vi "AB_Engine_InteropAssembly_ProtoDefined.vi"(0 "Parser":refnum<k24>, 1 "2011CompatibilityMode":bool, 5 "Build Interop Assembly for .NET 2.0":bool, 7 "ClassInfo":T3[](array[typedef]), 9 "ExportAssemblyVIinfo":T5[](array[typedef]), 11 "error in":errorcluster) -> (4 "Parser Out":refnum<k24>, 6 "ContainLVClass":bool, 8 "SetVIInformationArray":T2[](array[typedef]), 10 "SetLVCLassInformationArray":T1[](array[typedef]), 15 "error out":errorcluster)   [LabVIEW 2020]
uses:
  e:/builds/penguin/labview/branches/2020/dev/dist/resource/NationalInstruments.LabVIEW.Generator.dll
  resource/NationalInstruments.LabVIEW.Generator.dll
  <vilib>/AppBuilder/AB_InteropAssembly_DistVI_Proto_Info.ctl
  <vilib>/AppBuilder/IOStatus.ctl
  <vilib>/AppBuilder/AB_InteropAssembly_DistVI_Class_Info.ctl
  <vilib>/AppBuilder/AB_InteropAssembly_SetVIInformation.ctl
  <vilib>/AppBuilder/AB_InteropAssembly_SetLVClassInformation.ctl
panel:
  in  "SetLVCLassInformation":T1
  in  "SetVIInformation":T2
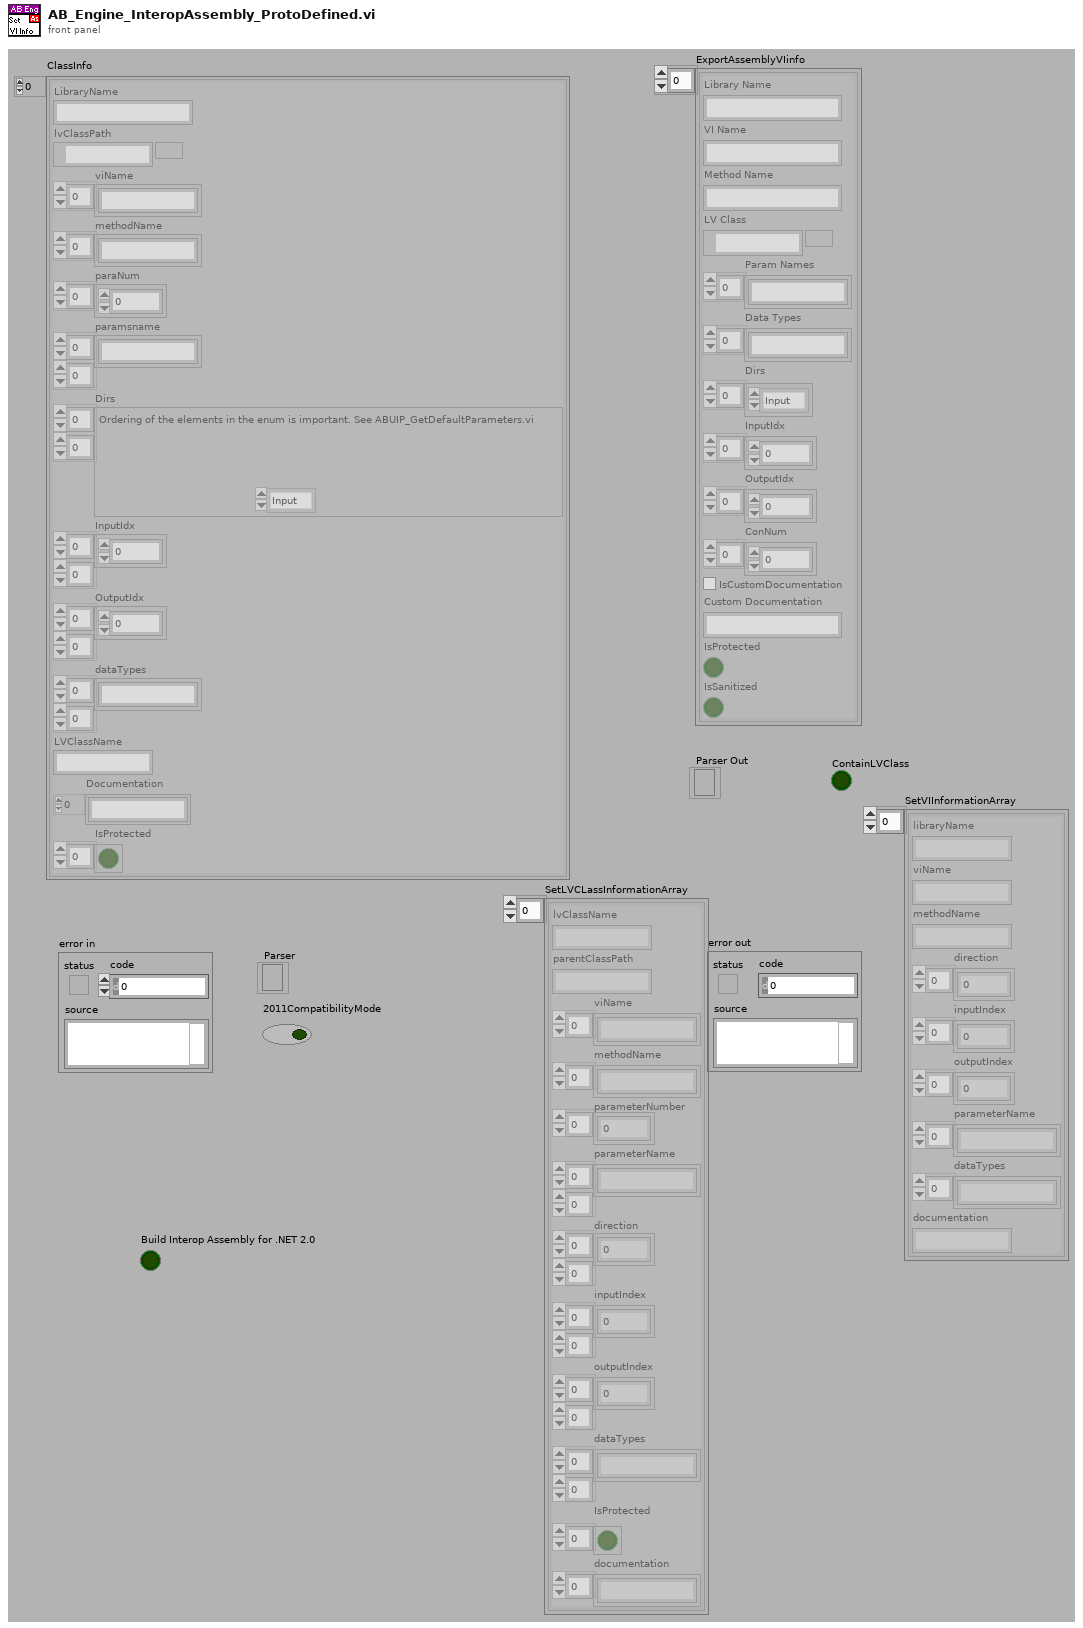
[diagram p1: front panel]
types:
  T1 = typedef "AB_InteropAssembly_SetLVClassInformation.ctl" = cluster{"lvClassName":string, "parentClassPath":string, "viName":string[], "methodName":string[], "parameterNumber":i32[], "parameterName":string[][], "direction":i32[][], "inputIndex":i32[][], "outputIndex":i32[][], "dataTypes":string[][], "IsProtected":bool[], "documentation":string[]}
  T2 = typedef "AB_InteropAssembly_SetVIInformation.ctl" = cluster{"libraryName":string, "viName":string, "methodName":string, "direction":i32[], "inputIndex":i32[], "outputIndex":i32[], "parameterName":string[], "dataTypes":string[], "documentation":string}
  T3 = typedef "AB_InteropAssembly_DistVI_Class_Info.ctl" = cluster{"LibraryName":string, "lvClassPath":path, "viName":string[], "methodName":string[], "paraNum":i32[], "paramsname":string[][], "Dirs":T4[][], "InputIdx":i32[][], "OutputIdx":i32[][], "dataTypes":string[][], "LVClassName":string, "Documentation":string[], "IsProtected":bool[]}
  T4 = typedef "IOStatus.ctl" = enum16{"Input", "Output", "Input/Output", "InputDeleted", "OutputDeleted", "IODeleted", "ErrorClusterIn", "ErrorClusterOut"}
  T5 = typedef "AB_InteropAssembly_DistVI_Proto_Info.ctl" = cluster{"Library Name":string, "VI Name":string, "Method Name":string, "LV Class":path, "Param Names":string[], "Data Types":string[], "Dirs":T4[], "InputIdx":i32[], "OutputIdx":i32[], "ConNum":i8[], "IsCustomDocumentation":bool, "Custom Documentation":string, "IsProtected":bool, "IsSanitized":bool}
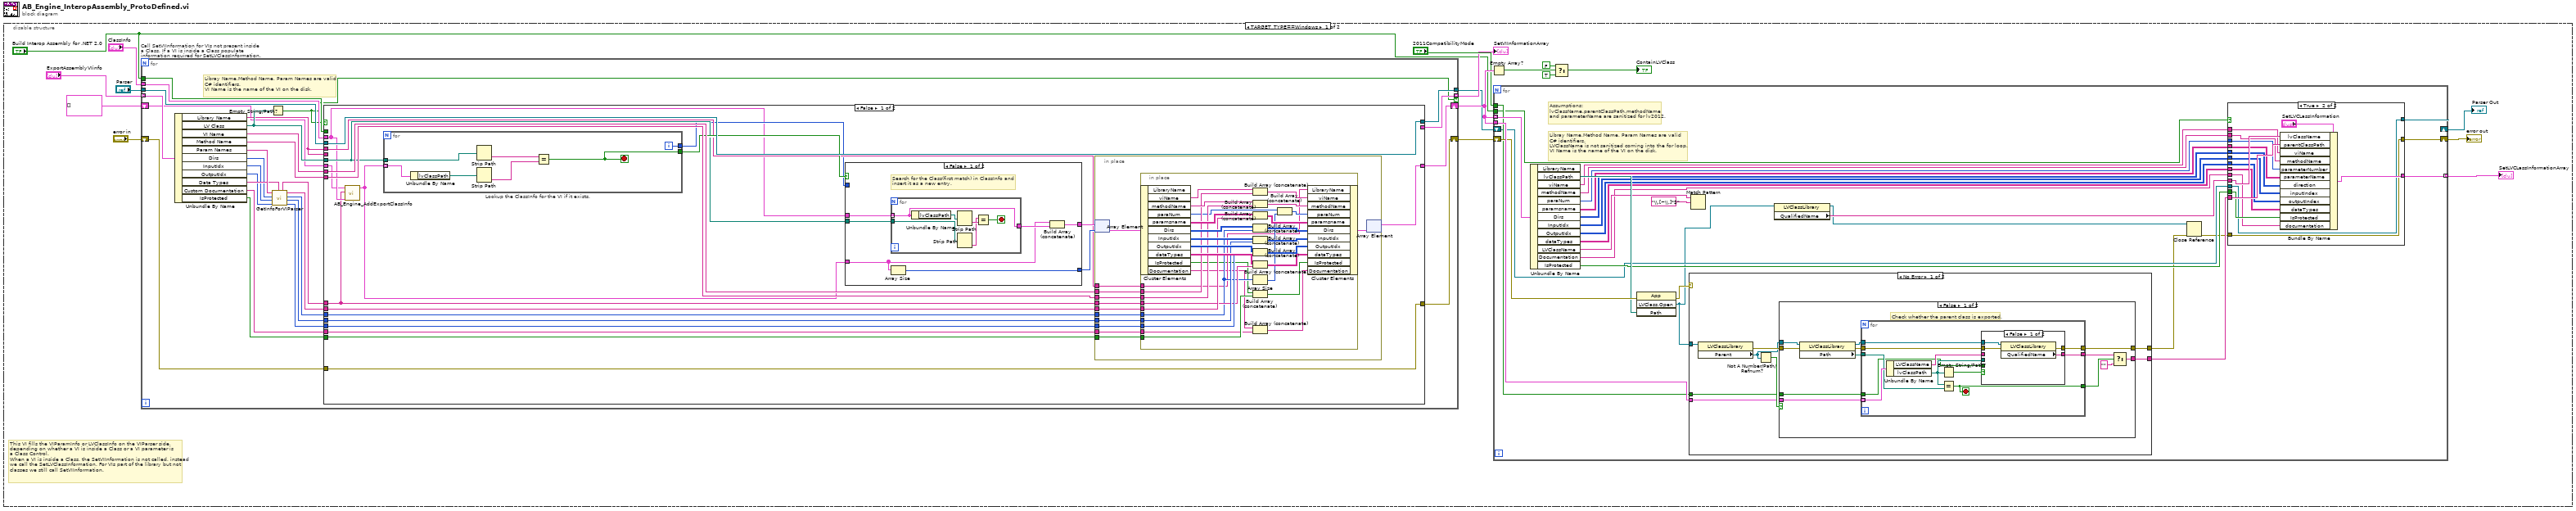
[diagram p0: block diagram]
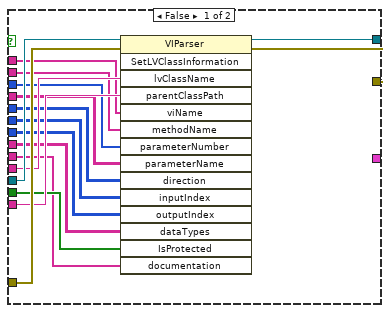
[diagram p2: hidden frame]
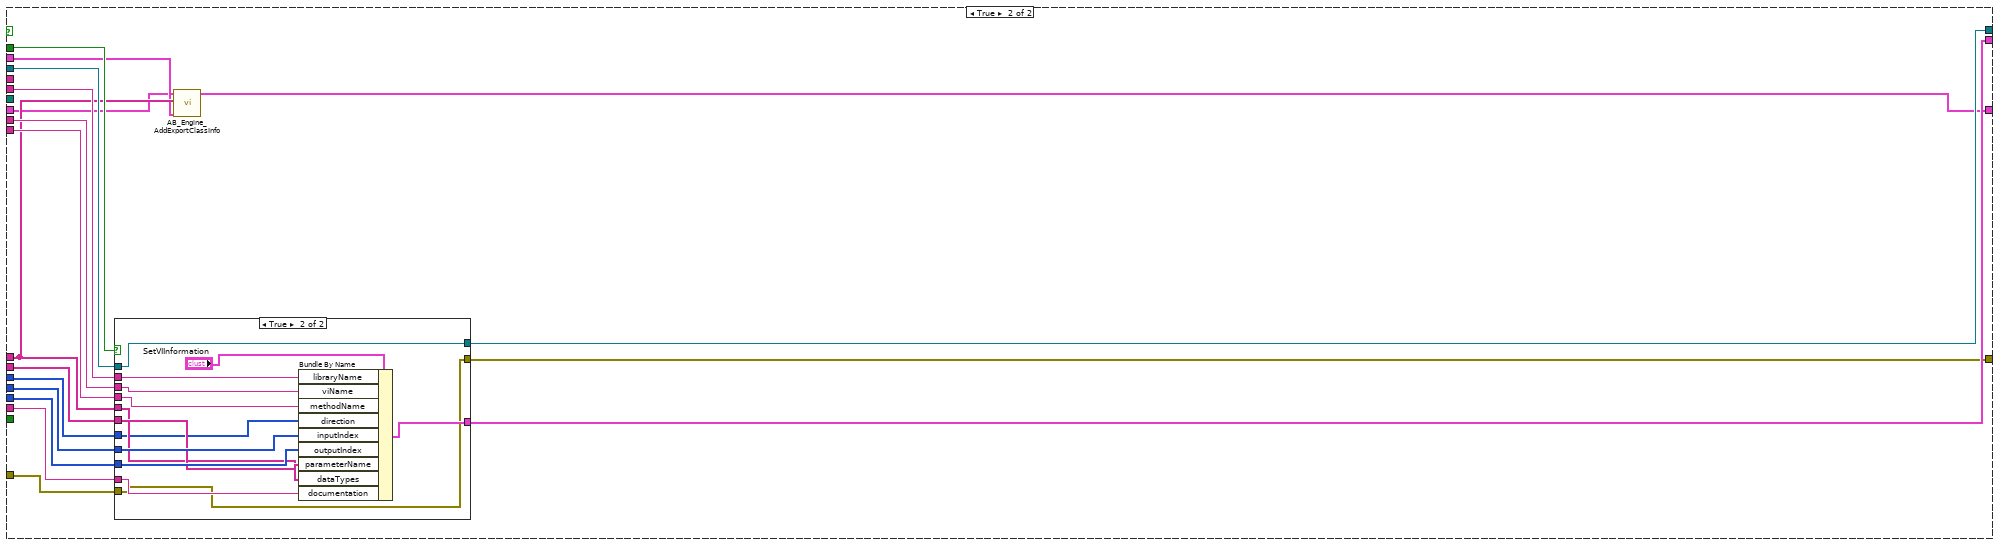
[diagram p7: hidden frame]
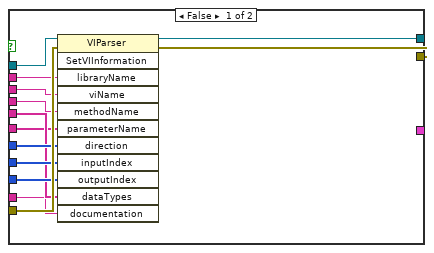
[diagram p8: hidden frame]
diagram:
  n1 = disable-structure shown="TARGET_TYPE==Windows" {
    frame condition #0 (active) {
      # "This VI fills the VIParamInfo or LVClassInfo on the VIParser side,\ndepending on whether a VI is inside a Class or a VI parameter is \na Class Control.\nWhen a VI is inside a Class, the SetVIInformation is not called, instead\nwe call the SetLVClassInformation. For VIs part of the library but not \nclasses we still call SetVIInformation."
      n2 = for "Call SetVIInformation for VIs not present inside a Class. If a VI is inside a Class populate information required for SetLVClassInformation." {
        tunnel: "ExportAssemblyVIinfo" -> [w144] mode=indexing
        tunnel: "Parser" -> [w143]
        shift-right: [w139] -> w15
        shift-left: "error in" -> [w140]
        shift-right: [w141] -> w9
        shift-left: T3[] [] -> [w118]
        tunnel: [w136] -> w2
        tunnel: "ClassInfo" -> [w135]
        tunnel: [w121] -> w4 mode=indexing if=w119
        tunnel: "Build Interop Assembly for .NET 2.0" -> [w120]
        # "Libray Name,Method Name, Param Names are valid\nC# identifiers.\nVI Name is the name of the VI on the disk."
        n3 = Unbundle By Name(w144) -> ("Library Name"=w134:string, "LV Class"=w137:path, "VI Name"=w138:string, "Method Name"=w142:string, "Param Names"=w132:string[], "Dirs"=w130:T4[], "InputIdx"=w129:i32[], "OutputIdx"=w128:i32[], "Data Types"=w131:string[], "Custom Documentation"=w133:string, "IsProtected"=w122:bool)
        n4 = Empty String/Path?(string/path=w137) -> (empty?=w119:bool)
        n5 = call <vilib>:"GetInfoForVIParser.vi"("Data Types"=w131, "OutputIdx"=w128, "InputIdx"=w129, "Dirs"=w130, "Param Names"=w132) -> ("OutputIdx Out"=w123:i32[], "InputIdx Out"=w124:i32[], "Dirs Out"=w126:T4[], "ParamNames Out"=w125:string[], "DataTypesOut"=w127:string[])
        n6 = case shown="False" w119 {
          tunnel: w143 -> [w157 w237]
          tunnel: w138 -> [w165 w244]
          tunnel: w142 -> [w164 w243]
          tunnel: w125 -> [w163 w239]
          tunnel: w126 -> [w162 w242]
          tunnel: w124 -> [w161 w241]
          tunnel: w123 -> [w160 w240]
          tunnel: w127 -> [w145 w233]
          tunnel: [w158 w234] -> w139
          tunnel: w118 -> [w146 w230]
          tunnel: w137 -> [w153 _]
          tunnel: [w159 w232] -> w141
          tunnel: w140 -> [w158 w236]
          tunnel: [w157 w235] -> w136
          tunnel: w135 -> [w147 w231]
          tunnel: w134 -> [w152 _]
          tunnel: w134 -> [_ w245]
          tunnel: w133 -> [w150 w238]
          tunnel: w122 -> [w151 _]
          tunnel: [_ w247] -> w121
          tunnel: w120 -> [_ w246]
          frame False {
            n7 = call <vilib>:"AB_Engine_AddExportClassInfo.vi"("ClassInfo"=w147, "DataTypes"=w145, "ExportClassInfo"=w146) -> ("ExportClassInfoOut"=w148:T3[])  [unwired: 8 in]
            n8 = for "Lookup the ClassInfo for the VI if it exists." {
              tunnel: w148 -> [w186] mode=indexing
              tunnel: w153 -> [w183]
              tunnel: [w184] -> w156
              tunnel: [w185] -> w149
              i -> [w185]
              stop <- w184 stop-if-true
              n9 = Unbundle By Name(w186) -> ("lvClassPath"=w181:path)
              n10 = Strip Path(path=w183) -> (name=w182:string)  [unwired: 1 out]
              n11 = Strip Path(path=w181) -> (name=w180:string)  [unwired: 1 out]
              n12 = Equal?(x=w182, y=w180) -> (x = y?=w184:bool)
            }
            n13 = case shown="False" w156 {
              tunnel: w148 -> [w167 w179]
              tunnel: [w171 w179] -> w155
              tunnel: [w166 w178] -> w154
              tunnel: w149 -> [_ w178]
              tunnel: w147 -> [w170 _]
              tunnel: w153 -> [w169 _]
              frame False {
                # "Search for the Class(first match) in ClassInfo and \ninsert it as a new entry."
                n14 = for {
                  tunnel: w170 -> [w172] mode=indexing
                  tunnel: w169 -> [w176]
                  tunnel: [w172] -> w168
                  stop <- w177 stop-if-true
                  n15 = Unbundle By Name(w172) -> ("lvClassPath"=w175:path)
                  n16 = Strip Path(path=w175) -> (name=w174:string)  [unwired: 1 out]
                  n17 = Strip Path(path=w176) -> (name=w173:string)  [unwired: 1 out]
                  n18 = Equal?(x=w173, y=w174) -> (x = y?=w177:bool)
                }
                n19 = Array Size(array=w167) -> (size(s)=w166:i32)
                n20 = Build Array (concatenate)(w167, w168) -> (w171:T3[])
              }
              frame True {
              }
            }
            n21 = in-place {
              in-place-border: w165 -> [w197]
              in-place-border: w164 -> [w196]
              in-place-border: w163 -> [w195]
              in-place-border: w162 -> [w194]
              in-place-border: w161 -> [w193]
              in-place-border: w160 -> [w192]
              in-place-border: w145 -> [w191]
              in-place-border: w152 -> [w189]
              in-place-border: w151 -> [w188]
              in-place-border: w150 -> [w187]
              n22 = in-place-array #1(w155, w154) -> (w198:T3)
              n23 = in-place {
                in-place-border: w197 -> [w211]
                in-place-border: w196 -> [w215]
                in-place-border: w195 -> [w214]
                in-place-border: w194 -> [w209]
                in-place-border: w193 -> [w213]
                in-place-border: w192 -> [w212]
                in-place-border: w191 -> [w210]
                in-place-border: w189 -> [w205]
                in-place-border: w188 -> [w203]
                in-place-border: w187 -> [w201]
                n24 = in-place-cluster #2(w198) -> ("viName"=w229:string[], "methodName"=w227:string[], "paraNum"=w208:i32[], "paramsname"=w225:string[][], "Dirs"=w223:T4[][], "InputIdx"=w221:i32[][], "OutputIdx"=w219:i32[][], "dataTypes"=w217:string[][], "IsProtected"=w204:bool[], "Documentation"=w200:string[])  [unwired: 1 out]
                n25 = Build Array (concatenate)(w229, w211) -> (w228:string[])
                n26 = Build Array (concatenate)(w227, w215) -> (w226:string[])
                n27 = Build Array (concatenate)(w225, w214) -> (w224:string[][])
                n28 = Build Array (concatenate)(w223, w209) -> (w222:T4[][])
                n29 = Build Array (concatenate)(w221, w213) -> (w220:i32[][])
                n30 = Build Array (concatenate)(w219, w212) -> (w218:i32[][])
                n31 = Build Array (concatenate)(w217, w210) -> (w216:string[][])
                n32 = Array Size(array=w209) -> (size(s)=w207:i32)
                n33 = Build Array (concatenate)(w204, w203) -> (w202:bool[])
                n34 = Build Array (concatenate)(w200, w201) -> (w199:string[])
                n35 = Build Array (concatenate)(w208, w207) -> (w206:i32[])
                n36 = in-place-cluster #2("LibraryName"=w205, "viName"=w228, "methodName"=w226, "paraNum"=w206, "paramsname"=w224, "Dirs"=w222, "InputIdx"=w220, "OutputIdx"=w218, "dataTypes"=w216, "IsProtected"=w202, "Documentation"=w199) -> (w190:T3)
              }
              n37 = in-place-array #1(w190) -> (w159:T3[])  [unwired: 1 out]
            }
          }
          frame True {
            n38 = case shown="True" w246 {
              tunnel: [_ w272] -> w247
              tunnel: w245 -> [w258 w271]
              tunnel: w244 -> [w257 w270]
              tunnel: w243 -> [w256 w269]
              tunnel: w242 -> [w255 w261]
              tunnel: w241 -> [w254 w268]
              tunnel: w240 -> [w253 w267]
              tunnel: w239 -> [w251 w266]
              tunnel: w233 -> [w252 w265]
              tunnel: w238 -> [w250 w264]
              tunnel: w237 -> [w260 w263]
              tunnel: w236 -> [w259 w262]
              tunnel: [w249 w263] -> w235
              tunnel: [w248 w262] -> w234
              frame False {
                n39 = invoke class="VIParser" method="SetVIInformation"(reference=w260, error in=w259, "libraryName"=w258, "viName"=w257, "methodName"=w256, "parameterName"=w251, "direction"=w255, "inputIndex"=w254, "outputIndex"=w253, "dataTypes"=w252, "documentation"=w250) -> (reference out=w249:refnum<k24>, error out=w248:errorcluster)  [unwired: 1 in, 10 out]
              }
              frame True {
                n40 = Bundle By Name(cluster="SetVIInformation", "libraryName"=w271, "viName"=w270, "methodName"=w269, "direction"=w261, "inputIndex"=w268, "outputIndex"=w267, "parameterName"=w266, "dataTypes"=w265, "documentation"=w264) -> (w272:T2)
              }
            }
            n41 = call <vilib>:"AB_Engine_AddExportClassInfo.vi"("ClassInfo"=w231, "DataTypes"=w233, "ExportClassInfo"=w230) -> ("ExportClassInfoOut"=w232:T3[])  [unwired: 8 in]
          }
        }
      }
      "SetVIInformationArray" <- w4
      n42 = Empty Array?(array=w9) -> (empty?=w14:bool)
      n43 = for {
        tunnel: w9 -> [w47] mode=indexing
        shift-right: [w25] -> w10
        shift-left: w15 -> [w45]
        tunnel: w9 -> [w46]
        shift-right: [w26] -> w8
        shift-left: w2 -> [w24]
        tunnel: "2011CompatibilityMode" -> [w40]
        tunnel: [w39] -> w3 mode=indexing
        tunnel: "Build Interop Assembly for .NET 2.0" -> [w27]
        # "Assumptions:\nlvClassName,parentClassPath,methodName\nand parameterName are sanitized for lv2012."
        # "Libray Name,Method Name, Param Names are valid\nC# identifiers.\nLVClassName is not sanitized coming into the for loop.\nVI Name is the name of the VI on the disk."
        n44 = Unbundle By Name(w47) -> ("lvClassPath"=w44:path, "viName"=w37:string[], "methodName"=w36:string[], "paraNum"=w35:i32[], "paramsname"=w34:string[][], "Dirs"=w33:T4[][], "InputIdx"=w32:i32[][], "OutputIdx"=w31:i32[][], "dataTypes"=w30:string[][], "LVClassName"=w41:string, "Documentation"=w28:string[], "IsProtected"=w29:bool[])  [unwired: 1 out]
        n45 = invoke class="App" method="LVClass.Open"(error in=w45, "Path"=w44) -> (error out=w43:errorcluster, "LVClass.Open"=w22:refnum<vi>)  [unwired: 2 in, 2 out]
        n46 = case shown="No Error" w43 {
          tunnel: w22 -> [w87 _]
          tunnel: [w86 _] -> w21
          tunnel: w46 -> [w82 _]
          tunnel: [w81 _] -> w38
          tunnel: w40 -> [w80 _]
          frame No Error {
            n47 = property class="LVClassLibrary"(reference=w87) -> (error out=w85:errorcluster, "Parent"=w84:refnum<vi>)  [unwired: 1 in, 1 out]
            n48 = Not A Number/Path/Refnum?(number/path/refnum=w84) -> (NaN/Path/Refnum?=w83:bool)
            n49 = case shown="False" w83 {
              tunnel: w84 -> [w98 _]
              tunnel: [w88 w117] -> w86
              tunnel: [w93 _] -> w81
              tunnel: w85 -> [w99 w117]
              tunnel: w82 -> [w97 _]
              tunnel: w80 -> [w91 _]
              frame False {
                # "Check whether the parent class is exported."
                n50 = property class="LVClassLibrary"(reference=w98, error in=w99) -> (reference out=w90:refnum<vi>, error out=w89:errorcluster, "Path"=w96:path)
                n51 = for {
                  tunnel: w97 -> [w110] mode=indexing
                  tunnel: w96 -> [w109]
                  tunnel: [w106] -> w95
                  tunnel: [w103] -> w94
                  tunnel: w91 -> [w104]
                  tunnel: w90 -> [w102]
                  tunnel: w89 -> [w101]
                  tunnel: [w100] -> w88
                  stop <- w106 stop-if-true
                  n52 = Unbundle By Name(w110) -> ("LVClassName"=w107:string, "lvClassPath"=w108:path)
                  n53 = Empty String/Path?(string/path=w108) -> (empty?=w105:bool)
                  n54 = Equal?(x=w108, y=w109) -> (x = y?=w106:bool)
                  n55 = case shown="False" w105 {
                    tunnel: w108 -> [_ _]
                    tunnel: w107 -> [_ w116]
                    tunnel: [w113 w116] -> w103
                    tunnel: w104 -> [_ _]
                    tunnel: w102 -> [w114 _]
                    tunnel: w101 -> [w112 w115]
                    tunnel: [w111 w115] -> w100
                    frame False {
                      n56 = property class="LVClassLibrary"(reference=w114, error in=w112) -> (error out=w111:errorcluster, "QualifiedName"=w113:string)  [unwired: 1 out]
                    }
                    frame True {
                    }
                  }
                }
                n57 = Select(t=w94, s=w95, f="") -> (s? t:f=w93:string)
              }
              frame True {
                # "LVClass does not have a parent Class."
              }
            }
          }
          frame Error {
            # "This LV Class is only used in VI's terminal"
          }
        }
        n58 = Match Pattern(string=w41, regular expression="\\.[~\\.]*$") -> ()  [unwired: 5 out]
        n59 = property class="LVClassLibrary"(reference=w22) -> (reference out=w19:refnum<vi>, "QualifiedName"=w23:string)  [unwired: 1 in, 1 out]
        n60 = Close Reference(reference=w19, error in (no error)=w21) -> (error out=w20:errorcluster)
        n61 = case shown="True" w27 {
          tunnel: [_ w78] -> w39
          tunnel: w23 -> [w59 w77]
          tunnel: w38 -> [w58 w76]
          tunnel: w37 -> [w57 w75]
          tunnel: w36 -> [w56 w74]
          tunnel: w35 -> [w55 w73]
          tunnel: w34 -> [w54 w72]
          tunnel: w33 -> [w53 w71]
          tunnel: w32 -> [w52 w70]
          tunnel: w31 -> [w51 w69]
          tunnel: w30 -> [w50 w68]
          tunnel: w29 -> [w49 w67]
          tunnel: w28 -> [w48 w64]
          tunnel: [w63 w66] -> w26
          tunnel: [w62 w65] -> w25
          tunnel: w24 -> [w61 w66]
          tunnel: w20 -> [w60 w65]
          frame False {
            n62 = invoke class="VIParser" method="SetLVClassInformation"(reference=w61, error in=w60, "lvClassName"=w59, "parentClassPath"=w58, "viName"=w57, "methodName"=w56, "parameterNumber"=w55, "parameterName"=w54, "direction"=w53, "inputIndex"=w52, "outputIndex"=w51, "dataTypes"=w50, "IsProtected"=w49, "documentation"=w48) -> (reference out=w63:refnum<k24>, error out=w62:errorcluster)  [unwired: 1 in, 13 out]
          }
          frame True {
            n63 = Bundle By Name(cluster="SetLVCLassInformation", "lvClassName"=w77, "parentClassPath"=w76, "viName"=w75, "methodName"=w74, "parameterNumber"=w73, "parameterName"=w72, "direction"=w71, "inputIndex"=w70, "outputIndex"=w69, "dataTypes"=w68, "IsProtected"=w67, "documentation"=w64) -> (w78:T1)
          }
        }
      }
      "error out" <- w10
      "Parser Out" <- w8
      "SetLVCLassInformationArray" <- w3
      n64 = Select(t=FALSE, s=w14, f=TRUE) -> (s? t:f=→"ContainLVClass":bool)
    }
    frame condition #1 {
    }
  }
